vi "TM Interfaces_Control_1.vi"() -> ()   [LabVIEW 2019]
uses:
  <instrlib>/niSwitch/niSwitch.llb/niSwitch Topologies.ctl
  <instrlib>/niSwitch/niSwitch.llb/niSwitch Relay Action.ctl
  <vilib>/DAQmx/write.llb/DAQmx Write (Analog DBL 1Chan 1Samp).vi
  <vilib>/DAQmx/read.llb/DAQmx Read (Analog 1D DBL 1Chan NSamp).vi
  <resource>/objmgr/daqmx.rc
  <vilib>/DAQmx/write.llb/DAQmx Write (Analog Wfm 1Chan NSamp).vi
  <vilib>/DAQmx/configure/timing.llb/DAQmx Timing (Implicit).vi
  <vilib>/DAQmx/create/channels.llb/DAQmx Create Channel (AO-Voltage-Basic).vi
  <vilib>/DAQmx/create/channels.llb/DAQmx Create Channel (AI-Voltage-Basic).vi
  <vilib>/DAQmx/create/channels.llb/DAQmx Create Channel (CO-Pulse Generation-Time).vi
  <vilib>/DAQmx/read.llb/DAQmx Read (Analog 2D DBL NChan NSamp).vi
  <vilib>/DAQmx/write.llb/DAQmx Write (Analog 2D DBL NChan NSamp).vi
  <instrlib>/niSwitch/niSwitch.llb/niSwitch Relay Position.ctl
panel:
  out "Waveform Chart":cluster{"Waveform":dbl, "Waveform":dbl}(graph)
  in  "data":dbl[][](array[numeric]) min=0.0 max=5.12 format="%0.2f"
  out "Waveform Chart 2":cluster{"Waveform":dbl, "Waveform":dbl}(graph)
  in  "TM Interface Name":string
  in  "Value":string
  out "Pulse Generating?":bool
  out "Angular Velocity Telemetry":dbl
  out "Ø Sweep Chart":dbl(graph)
  out "Ø(n)":dbl
  out "2pi/18":dbl
  out "Ø(n-1)":dbl
  out "^Ø":dbl
  out "Position of Relay":T1=10 caption="position" items=["Open"=10, "Closed"=11]
  out "Direction Voltage Generate?":bool
  out "Rotation of Direction Voltage Value":dbl
  out "Direction of Rotation":string
  out "Iteration of RW Direction of Rotation TM Model":i32
  out "Rotation of Direction Voltage Acquire":dbl[](graph)
  out "RW Dir Voltage Acquire?":bool
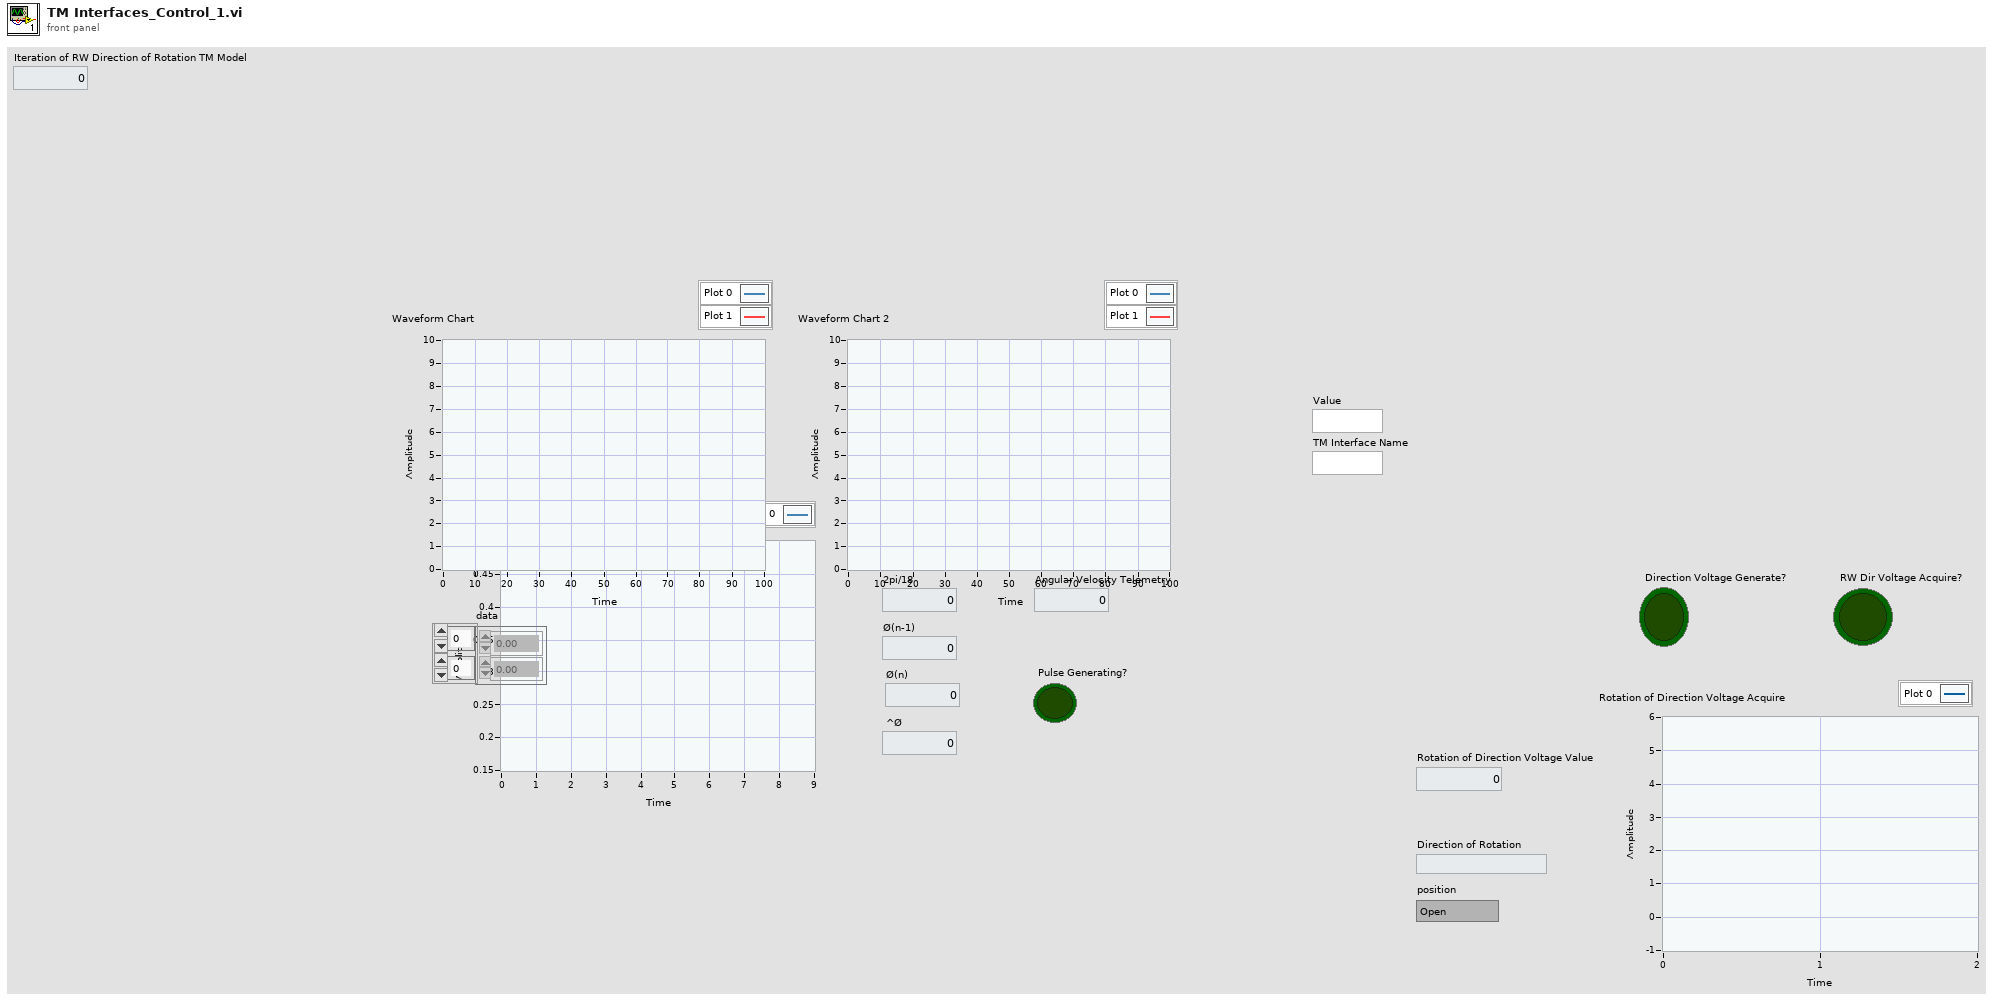
[diagram p1: front panel]
types:
  T1 = typedef "niSwitch Relay Position.ctl" = i32
  T2 = typedef "niSwitch Topologies.ctl" = string
  T3 = typedef "niSwitch Relay Action.ctl" = i32
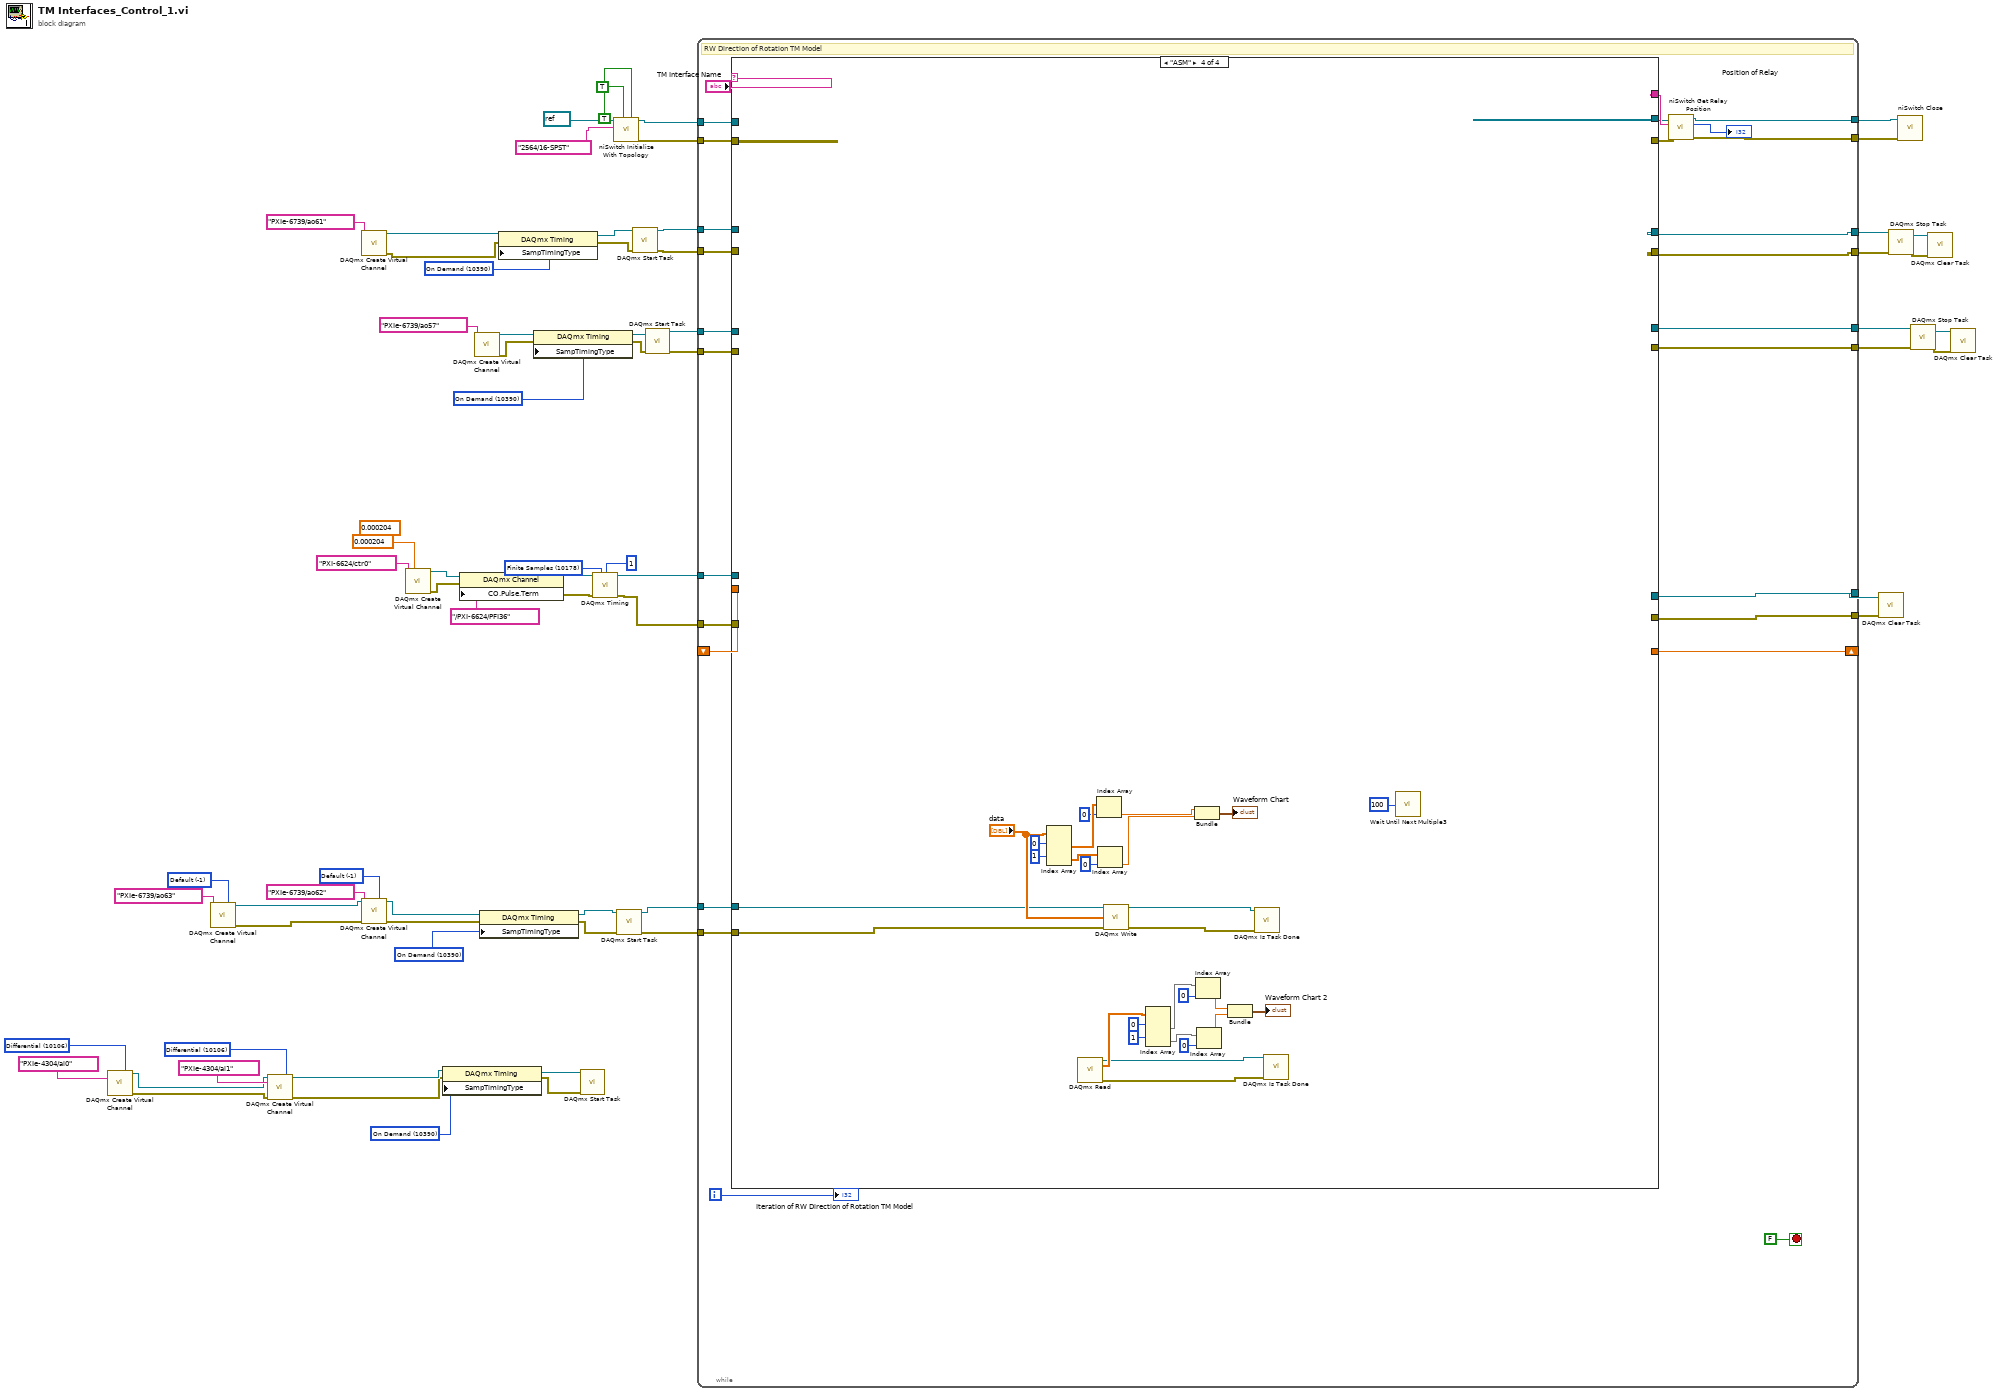
[diagram p0: block diagram]
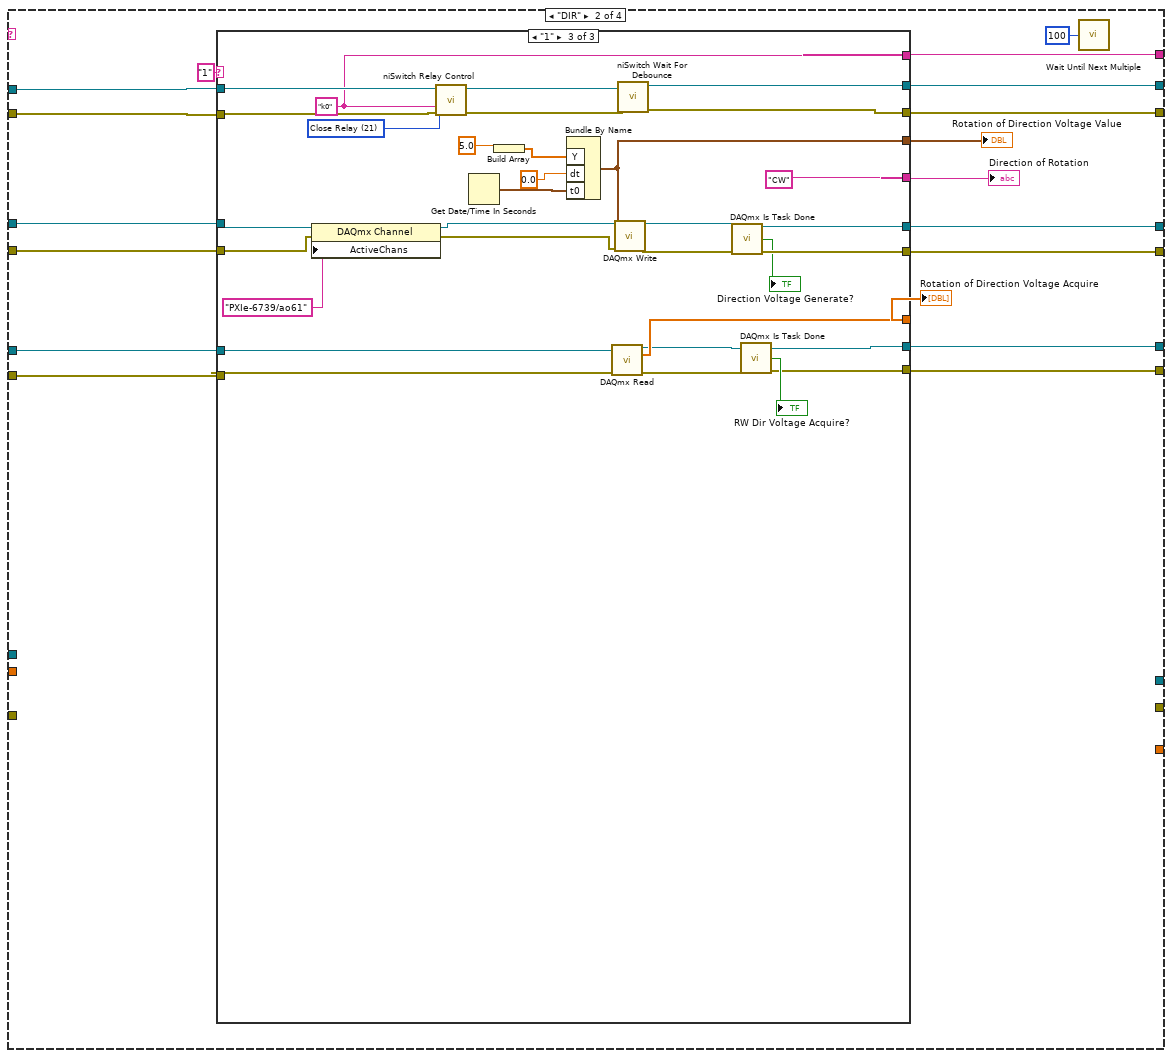
[diagram p3: hidden frame]
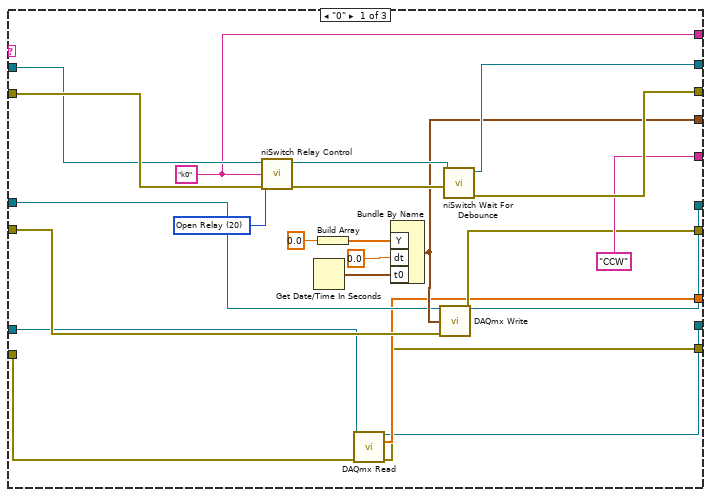
[diagram p4: hidden frame]
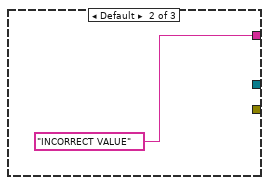
[diagram p5: hidden frame]
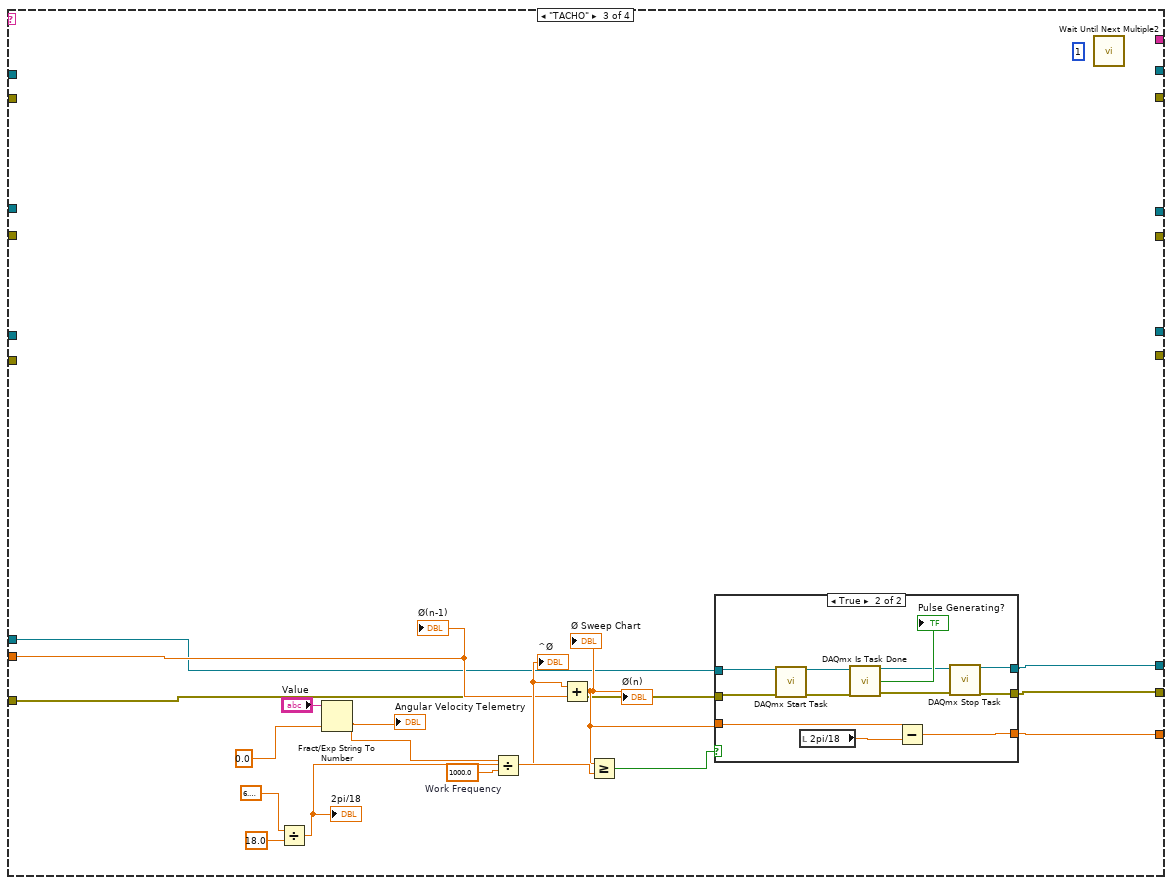
[diagram p6: hidden frame]
diagram:
  w1 = 10390 items=["Sample Clock"=10388, "Burst Handshake"=12548, "Handshake"=10389, "Implicit"=10451, "On Demand"=10390, "Change Detection"=12504, "Pipelined Sample Clock"=14668] ("SampTimingType")
  w6 = 10106 items=["Default"=-1, "RSE"=10083, "NRSE"=10078, "Differential"=10106, "Pseudodifferential"=12529] ("input terminal configuration")
  w9 = 10106 items=["Default"=-1, "RSE"=10083, "NRSE"=10078, "Differential"=10106, "Pseudodifferential"=12529] ("input terminal configuration")
  w20 = -1 items=["Default"=-1, "RSE"=10083, "Differential"=10106, "Pseudodifferential"=12529] ("output terminal configuration")
  w14 = 10390 items=["Sample Clock"=10388, "Burst Handshake"=12548, "Handshake"=10389, "Implicit"=10451, "On Demand"=10390, "Change Detection"=12504, "Pipelined Sample Clock"=14668] ("SampTimingType")
  w23 = -1 items=["Default"=-1, "RSE"=10083, "Differential"=10106, "Pseudodifferential"=12529] ("output terminal configuration")
  w43 = 10178 items=["Finite Samples"=10178, "Continuous Samples"=10123, "Hardware Timed Single Point"=12522] ("sample mode")
  (unwired) 0.000204 ("low time")
  w51 = 10390 items=["Sample Clock"=10388, "Burst Handshake"=12548, "Handshake"=10389, "Implicit"=10451, "On Demand"=10390, "Change Detection"=12504, "Pipelined Sample Clock"=14668] ("SampTimingType")
  w59 = 10390 items=["Sample Clock"=10388, "Burst Handshake"=12548, "Handshake"=10389, "Implicit"=10451, "On Demand"=10390, "Change Detection"=12504, "Pipelined Sample Clock"=14668] ("SampTimingType")
  n1 = call-poly <vilib>:"DAQmx Create Virtual Channel.vi"("input terminal configuration"=w6, "physical channels"=tag "PXIe-4304/ai0") -> ("task out"=w5:refnum<k21>, "error out"=w4:errorcluster)  [unwired: 12 in]
  n2 = call-poly <vilib>:"DAQmx Create Virtual Channel.vi"("output terminal configuration"=w23, "physical channels"=tag "PXIe-6739/ao63") -> ("task out"=w18:refnum<k21>, "error out"=w17:errorcluster)  [unwired: 12 in]
  n3 = call-poly <vilib>:"DAQmx Create Virtual Channel.vi"("task in"=w5, "input terminal configuration"=w9, "physical channels"=tag "PXIe-4304/ai1", "error in"=w4) -> ("task out"=w3:refnum<k21>, "error out"=w2:errorcluster)  [unwired: 10 in]
  n4 = call-poly <vilib>:"DAQmx Create Virtual Channel.vi"("physical channels"=tag "PXIe-6739/ao61") -> ("task out"=w28:refnum<k21>, "error out"=w27:errorcluster)  [unwired: 13 in]
  n5 = call-poly <vilib>:"DAQmx Create Virtual Channel.vi"("task in"=w18, "output terminal configuration"=w20, "physical channels"=tag "PXIe-6739/ao62", "error in"=w17) -> ("task out"=w16:refnum<k21>, "error out"=w15:errorcluster)  [unwired: 10 in]
  n6 = call-poly <vilib>:"DAQmx Create Virtual Channel.vi"("high time"=0.000204, "counter"=tag "PXI-6624/ctr0") -> ("task out"=w38:refnum<k21>, "error out"=w39:errorcluster)  [unwired: 12 in]
  n7 = property class="DAQmx Timing"(reference=w3, error in=w2, "SampTimingType"=w1) -> (reference out=w11:refnum<k21>, error out=w10:errorcluster)
  n8 = property class="DAQmx Channel"(reference=w38, error in=w39, "CO.Pulse.Term"=tag "/PXI-6624/PFI36") -> (reference out=w45:refnum<k21>, error out=w44:errorcluster)
  n9 = call-poly <vilib>:"DAQmx Create Virtual Channel.vi"("physical channels"=tag "PXIe-6739/ao57") -> ("task out"=w55:refnum<k21>, "error out"=w54:errorcluster)  [unwired: 13 in]
  n10 = property class="DAQmx Timing"(reference=w16, error in=w15, "SampTimingType"=w14) -> (reference out=w22:refnum<k21>, error out=w21:errorcluster)
  n11 = property class="DAQmx Timing"(reference=w28, error in=w27, "SampTimingType"=w59) -> (reference out=w31:refnum<k21>, error out=w30:errorcluster)
  n12 = property class="DAQmx Timing"(reference=w55, error in=w54, "SampTimingType"=w51) -> (reference out=w53:refnum<k21>, error out=w52:errorcluster)
  n13 = call <vilib>:"DAQmx Start Task.vi"("task/channels in"=w11, "error in"=w10) -> ()  [unwired: 12 in, 2 out]
  n14 = call-poly <vilib>:"DAQmx Timing.vi"("task/channels in"=w45, "sample mode"=w43, "samples per channel"=1, "error in"=w44) -> ("task out"=w35:refnum<k21>, "error out"=w34:errorcluster)  [unwired: 10 in]
  n15 = call <instrlib>:"niSwitch Initialize With Topology.vi"("simulate (boolean value)"=TRUE, "reset device (boolean value)"=TRUE, "topology name"=T2 "2564/16-SPST", "resource name"=refnum<k15> refnum) -> ("error out"=w63:errorcluster, "instrument handle out"=w62:refnum<k15>)  [unwired: 1 in, 5 out]
  n16 = call <vilib>:"DAQmx Start Task.vi"("task/channels in"=w22, "error in"=w21) -> ("task out"=w13:refnum<k21>, "error out"=w12:errorcluster)  [unwired: 12 in]
  n17 = call <vilib>:"DAQmx Start Task.vi"("task/channels in"=w31, "error in"=w30) -> ("task out"=w33:refnum<k21>, "error out"=w32:errorcluster)  [unwired: 12 in]
  n18 = call <vilib>:"DAQmx Start Task.vi"("task/channels in"=w53, "error in"=w52) -> ("task out"=w50:refnum<k21>, "error out"=w49:errorcluster)  [unwired: 12 in]
  n19 = while {
    tunnel: w33 -> [w88]
    tunnel: w32 -> [w87]
    tunnel: w63 -> [w96]
    tunnel: [w93] -> w60
    tunnel: w62 -> [w95]
    tunnel: [w94] -> w61
    tunnel: [w86] -> w58
    tunnel: [w85] -> w57
    tunnel: w50 -> [w82]
    tunnel: w49 -> [w81]
    tunnel: [w72] -> w37
    tunnel: [w80] -> w36
    shift-right: [w79] -> _
    shift-left: _ -> [w78]
    tunnel: w35 -> [w77]
    tunnel: w34 -> [w76]
    tunnel: [w74] -> w26
    tunnel: [w73] -> w25
    tunnel: w13 -> [w71]
    tunnel: w12 -> [w70]
    i -> [w83]
    stop <- FALSE stop-if-true
    # "RW Direction of Rotation TM Model"
    n20 = case shown="\"ASM\"" "TM Interface Name" {
      tunnel: [_ w114 _ _] -> w92
      tunnel: [_ w113 _ _] -> w91
      tunnel: [_ w112 _ _] -> w90
      tunnel: w96 -> [_ w111 _ _]
      tunnel: w95 -> [_ w110 _ _]
      tunnel: w88 -> [_ w109 _ _]
      tunnel: w87 -> [_ w108 _ _]
      tunnel: [_ w107 _ _] -> w86
      tunnel: [_ w106 _ _] -> w85
      tunnel: w82 -> [_ w105 _ _]
      tunnel: w81 -> [_ w104 _ _]
      tunnel: [_ _ w176 _] -> w72
      tunnel: [_ _ w175 _] -> w80
      tunnel: [_ _ w174 _] -> w79
      tunnel: w78 -> [_ _ w173 _]
      tunnel: w77 -> [_ _ w172 _]
      tunnel: w76 -> [_ _ w171 _]
      tunnel: [_ w99 _ _] -> w74
      tunnel: [_ w98 _ _] -> w73
      tunnel: w71 -> [_ _ _ w200]
      tunnel: w70 -> [_ _ _ w199]
      frame "", Default {
      }
      frame "DIR" {
        n21 = case shown="\"1\"" "1" {
          tunnel: w111 -> [w135 _ w166]
          tunnel: w110 -> [w134 _ w167]
          tunnel: [w130 _ w164] -> w114
          tunnel: [w132 _ w163] -> w113
          tunnel: [w131 _ w162] -> w112
          tunnel: ["CCW" ("String") "INCORRECT VALUE" ("String") "CW" ("String")] -> w101
          tunnel: w109 -> [w123 _ w145]
          tunnel: w108 -> [w122 _ w144]
          tunnel: [w121 _ w154] -> w107
          tunnel: [w120 _ w153] -> w106
          tunnel: [w124 _ w151] -> w102
          tunnel: w105 -> [w119 _ w150]
          tunnel: w104 -> [w118 _ w149]
          tunnel: [w116 _ w147] -> w99
          tunnel: [w115 _ w139] -> w98
          tunnel: [w117 _ w148] -> w100
          frame "0" {
            w133 = T3 20 items=["Open Relay"=20, "Close Relay"=21] ("relay action (Close Relay)")
            w132 = "k0" ("relay names")
            n22 = call <instrlib>:"niSwitch Relay Control.vi"("error in (no error)"=w135, "relay action (Close Relay)"=w133, "relay names"=w132, "instrument handle"=w134) -> ("error out"=w137:errorcluster, "instrument handle out"=w136:refnum<k15>)  [unwired: 6 out]
            n23 = Get Date/Time In Seconds() -> (seconds since 1Jan1904=w128:timestamp)
            n24 = Build Array "Build Array"(0.0 ("element")) -> (w129:dbl[])
            n25 = call-poly <vilib>:"DAQmx Read.vi"("task/channels in"=w119, "error in"=w118) -> ("task out"=w116:refnum<k21>, "data"=w117:dbl[], "error out"=w115:errorcluster)  [unwired: 11 in]
            n26 = Bundle By Name("Y"=w129, "dt"=0.0 ("element"), "t0"=w128) -> (w124:waveform(dbl))  [unwired: 1 in]
            n27 = call-poly <vilib>:"DAQmx Write.vi"("task/channels in"=w123, "data"=w124, "error in"=w122) -> ("task out"=w121:refnum<k21>, "error out"=w120:errorcluster)  [unwired: 10 in, 1 out]
            n28 = call <instrlib>:"niSwitch Wait For Debounce.vi"("error in (no error)"=w137, "instrument handle"=w136) -> ("error out"=w130:errorcluster, "instrument handle out"=w131:refnum<k15>)  [unwired: 1 in, 7 out]
          }
          frame Default {
          }
          frame "1" {
            w165 = T3 21 items=["Open Relay"=20, "Close Relay"=21] ("relay action (Close Relay)")
            w163 = "k0" ("relay names")
            n29 = property class="DAQmx Channel"(reference=w145, error in=w144, "ActiveChans"="PXIe-6739/ao61") -> (reference out=w143:refnum<k21>, error out=w142:errorcluster)
            n30 = call <instrlib>:"niSwitch Relay Control.vi"("error in (no error)"=w166, "relay action (Close Relay)"=w165, "relay names"=w163, "instrument handle"=w167) -> ("error out"=w168:errorcluster, "instrument handle out"=w169:refnum<k15>)  [unwired: 6 out]
            n31 = Get Date/Time In Seconds() -> (seconds since 1Jan1904=w160:timestamp)
            n32 = Build Array "Build Array"(5.0 ("element")) -> (w161:dbl[])
            n33 = Bundle By Name("Y"=w161, "dt"=0.0 ("element"), "t0"=w160) -> (w151:waveform(dbl))  [unwired: 1 in]
            n34 = call-poly <vilib>:"DAQmx Read.vi"("task/channels in"=w150, "error in"=w149) -> ("task out"=w147:refnum<k21>, "data"=w148:dbl[], "error out"=w140:errorcluster)  [unwired: 11 in]
            n35 = call-poly <vilib>:"DAQmx Write.vi"("task/channels in"=w143, "data"=w151, "error in"=w142) -> ("task out"=w156:refnum<k21>, "error out"=w155:errorcluster)  [unwired: 10 in, 1 out]
            n36 = call <instrlib>:"niSwitch Wait For Debounce.vi"("error in (no error)"=w168, "instrument handle"=w169) -> ("error out"=w164:errorcluster, "instrument handle out"=w162:refnum<k15>)  [unwired: 1 in, 7 out]
            n37 = call <vilib>:"DAQmx Is Task Done.vi"("task/channels in"=w156, "error in"=w155) -> ("task out"=w154:refnum<k21>, "task done?"=→"Direction Voltage Generate?":bool, "error out"=w153:errorcluster)  [unwired: 11 in]
            n38 = call <vilib>:"DAQmx Is Task Done.vi"("error in"=w140) -> ("task done?"=→"RW Dir Voltage Acquire?":bool, "error out"=w139:errorcluster)  [unwired: 12 in, 1 out]
          }
        }
        "Rotation of Direction Voltage Value" <- w102
        "Direction of Rotation" <- w101
        "Rotation of Direction Voltage Acquire" <- w100
        n39 = call "Wait Until Next Multiple"("Count(mSec)"=u32 100) -> ()  [unwired: 1 out]
      }
      frame "TACHO" {
        (unwired) u32 1 ("Count(mSec)")
        w182 = 1000.0  # Work Frequency
        n40 = Divide(x=6.283185307179586, y=18.0) -> (x/y=w185:dbl)
        "2pi/18" <- w185
        n41 = Fract/Exp String To Number(string="Value", default (0 dbl)=0.0) -> (number=w178:dbl)  [unwired: 2 in, 1 out]
        "Angular Velocity Telemetry" <- w178
        n42 = Divide(x=w178, y=w182) -> (x/y=w181:dbl)
        "^Ø" <- w181
        n43 = Add(x=w181, y=w173) -> (x+y=w180:dbl)
        "Ø(n)" <- w180
        "Ø Sweep Chart" <- w180
        n44 = Greater Or Equal?(x=w180, y=w185) -> (x >= y?=w177:bool)
        n45 = case shown="True" w177 {
          tunnel: w180 -> [w186 w197]
          tunnel: [w186 w196] -> w174
          tunnel: w172 -> [_ w194]
          tunnel: w171 -> [_ w191]
          tunnel: [_ w188] -> w176
          tunnel: [_ w187] -> w175
          frame False {
          }
          frame True {
            n46 = call <vilib>:"DAQmx Start Task.vi"("task/channels in"=w194, "error in"=w191) -> ("task out"=w193:refnum<k21>, "error out"=w192:errorcluster)  [unwired: 12 in]
            n47 = local read "2pi/18"() -> (w198:dbl)
            n48 = call <vilib>:"DAQmx Is Task Done.vi"("task/channels in"=w193, "error in"=w192) -> ("task out"=w190:refnum<k21>, "task done?"=→"Pulse Generating?":bool, "error out"=w189:errorcluster)  [unwired: 11 in]
            n49 = Subtract(x=w197, y=w198) -> (x-y=w196:dbl)
            n50 = call <vilib>:"DAQmx Stop Task.vi"("task/channels in"=w190, "error in"=w189) -> ("task out"=w188:refnum<k21>, "error out"=w187:errorcluster)  [unwired: 12 in]
          }
        }
        n51 = call "Wait Until Next Multiple2"() -> ()  [unwired: 1 in, 1 out]
        "Ø(n-1)" <- w173
      }
      frame "ASM" {
        n52 = Index Array(array="data", index (row) #1=0 ("index (row)"), index (row) #2=1 ("index (row)")) -> (element #1=w211:dbl[], element #2=w208:dbl[])  [unwired: 2 in]
        n53 = call-poly <vilib>:"DAQmx Read.vi"() -> ("task out"=w202:refnum<k21>, "data"=w221:dbl[][], "error out"=w201:errorcluster)  [unwired: 13 in]
        n54 = Index Array(array=w211, index=0) -> (element=w209:dbl)
        n55 = Index Array(array=w208, index=0) -> (element=w206:dbl)
        n56 = call-poly <vilib>:"DAQmx Write.vi"("task/channels in"=w200, "data"="data", "error in"=w199) -> ("task out"=w204:refnum<k21>, "error out"=w203:errorcluster)  [unwired: 10 in, 1 out]
        n57 = Index Array(array=w221, index (row) #1=0 ("index (row)"), index (row) #2=1 ("index (row)")) -> (element #1=w220:dbl[], element #2=w219:dbl[])  [unwired: 2 in]
        n58 = Bundle("Waveform"=w209, "Waveform"=w206) -> (→"Waveform Chart":cluster{"Waveform":dbl, "Waveform":dbl})  [unwired: 1 in]
        n59 = Index Array(array=w220, index=0) -> (element=w217:dbl)
        n60 = Index Array(array=w219, index=0) -> (element=w216:dbl)
        n61 = Bundle("Waveform"=w217, "Waveform"=w216) -> (→"Waveform Chart 2":cluster{"Waveform":dbl, "Waveform":dbl})  [unwired: 1 in]
        n62 = call <vilib>:"DAQmx Is Task Done.vi"("task/channels in"=w204, "error in"=w203) -> ()  [unwired: 11 in, 3 out]
        n63 = call <vilib>:"DAQmx Is Task Done.vi"("task/channels in"=w202, "error in"=w201) -> ()  [unwired: 11 in, 3 out]
        n64 = call "Wait Until Next Multiple3"("Count(mSec)"=u32 100) -> ()  [unwired: 1 out]
      }
    }
    n65 = call <instrlib>:"niSwitch Get Relay Position.vi"("error in (no error)"=w92, "relay name"=w91, "instrument handle"=w90) -> ("error out"=w93:errorcluster, "position"=→"Position of Relay":T1, "instrument handle out"=w94:refnum<k15>)  [unwired: 6 in]
    "Iteration of RW Direction of Rotation TM Model" <- w83
  }
  n66 = call <vilib>:"DAQmx Clear Task.vi"("task in"=w37, "error in"=w36) -> ()  [unwired: 13 in, 1 out]
  n67 = call <vilib>:"DAQmx Stop Task.vi"("task/channels in"=w58, "error in"=w57) -> ("task out"=w69:refnum<k21>, "error out"=w68:errorcluster)  [unwired: 12 in]
  n68 = call <instrlib>:"niSwitch Close.vi"("error in (no error)"=w60, "instrument handle"=w61) -> ()  [unwired: 10 out]
  n69 = call <vilib>:"DAQmx Stop Task.vi"("task/channels in"=w26, "error in"=w25) -> ("task out"=w48:refnum<k21>, "error out"=w47:errorcluster)  [unwired: 12 in]
  n70 = call <vilib>:"DAQmx Clear Task.vi"("task in"=w69, "error in"=w68) -> ()  [unwired: 13 in, 1 out]
  n71 = call <vilib>:"DAQmx Clear Task.vi"("task in"=w48, "error in"=w47) -> ()  [unwired: 13 in, 1 out]
